vi "NE-50X Single Run Edited.vi"() -> ()   [LabVIEW 2020]
doc: "This VI allows to perform a single run pumping mode : the pump run continuously until the user decide to stop, reverse or pause it."
uses:
  <vilib>/Utility/error.llb/DialogType.ctl
panel:
  in  "Extrusions to Do":i32
  out "Extrusions":i32
  in  "Volume":dbl
  out "Firmware Version":string
  out "Firmware Version":string
  in  "Secondary Pump Address":i32 format="%0#.0f"
  in  "Master Pump Address":i32 format="%0#.0f"
  out "Tank 2":dbl(slide)
  out "x+y":i32
  out "Tank":dbl(slide)
  in  "PAUSE 2":bool
  in  "Baud Rate (19200)":u32(ring)=19200 items=["19200"=19200, "9600"=9600, "2400"=2400, "1200"=1200, "300"=300]
  in  "VISA resource name":refnum<visa-resource-name>="ASRL1::INSTR"
  in  "PAUSE":bool
  in  "RUN":bool
  in  "STOP":bool
  in  "Audible Alarms":bool=TRUE
  in  "Flow rate\nSee below to enter a right value for flow rate":dbl=0.5 format="%.3f"
  in  "Units":i32(ring) items=["microlitters per minute (µL/min)", "microlitters per hour (µL/hr)", "milliliters per minute (mL/min)", "milliliters per hour (mL/hr)"]
  in  "Initial Direction":u16(ring) items=["Infuse", "Withdraw"]
  in  "Syringe Inside Diameter (19.58 mm)\nIf diameter is upper than 14.00 mm : Volume units are mL\nIf diameter is lower than 14.00 mm : Volume units are µL":dbl=19.58 min=0.1 max=50.0 step=0.01 format="%#_4g"
  out "Status":T1
  out "Volume Dispense":string
  # "Current Status"
  # "Configuration Settings"
  # "Pump System Config"
  # "mm"
  # "RS-232 Setup"
  # "Pump Control"
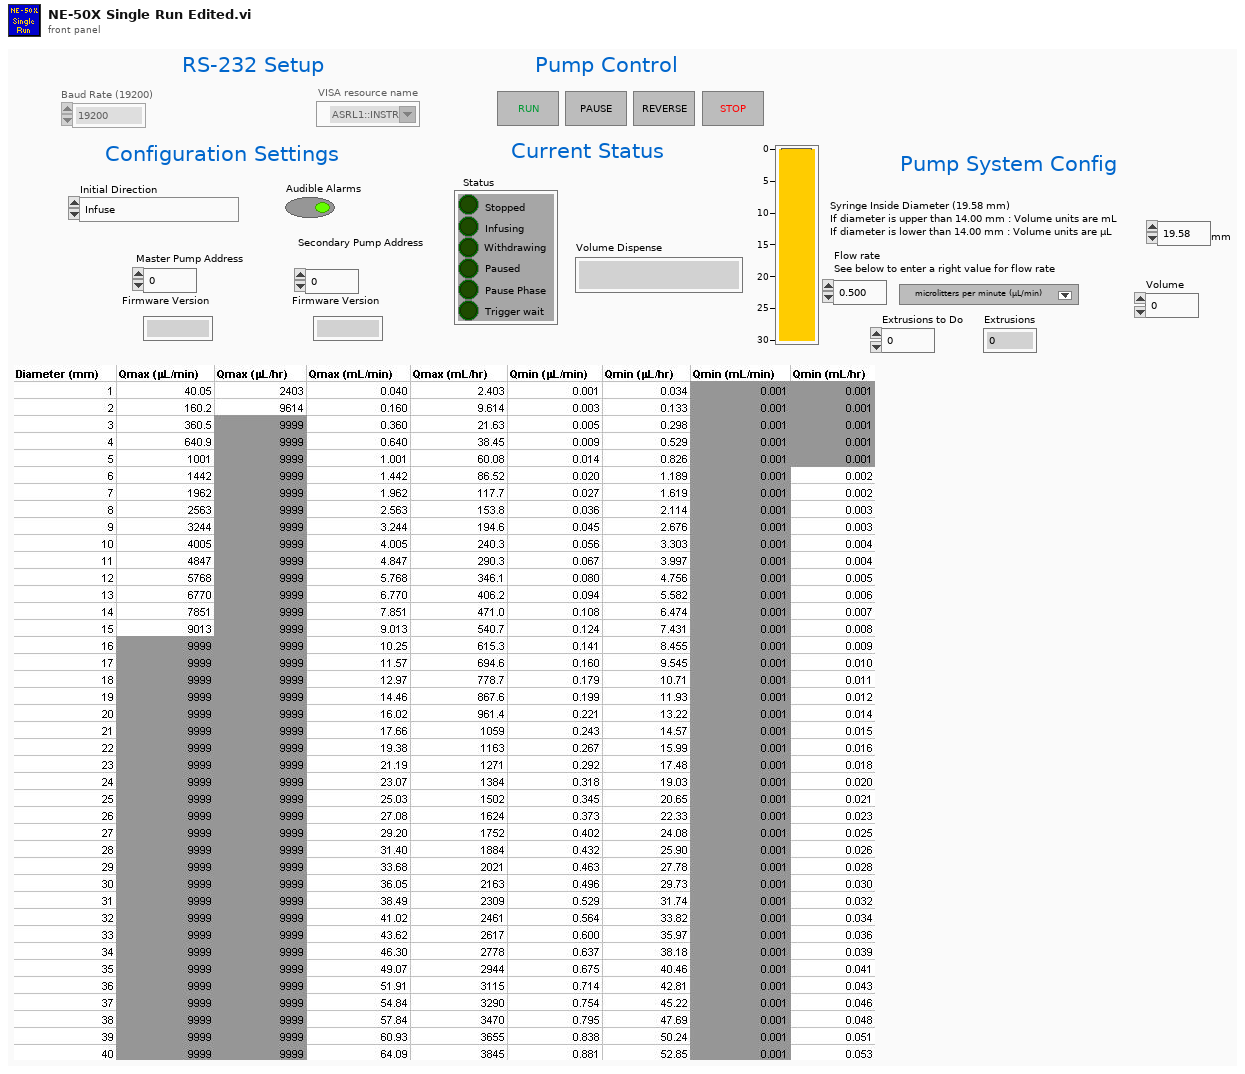
[diagram p1: front panel]
types:
  T1 = cluster{"Stopped":bool, "Infusing":bool, "Withdrawing":bool, "Paused":bool, "Pause Phase":bool, "Trigger wait":bool}
  T2 = typedef "DialogType.ctl" = u16
  T3 = cluster{"0=off\n1=on":u16, "Numbers of beeps\n0=continuously":dbl}
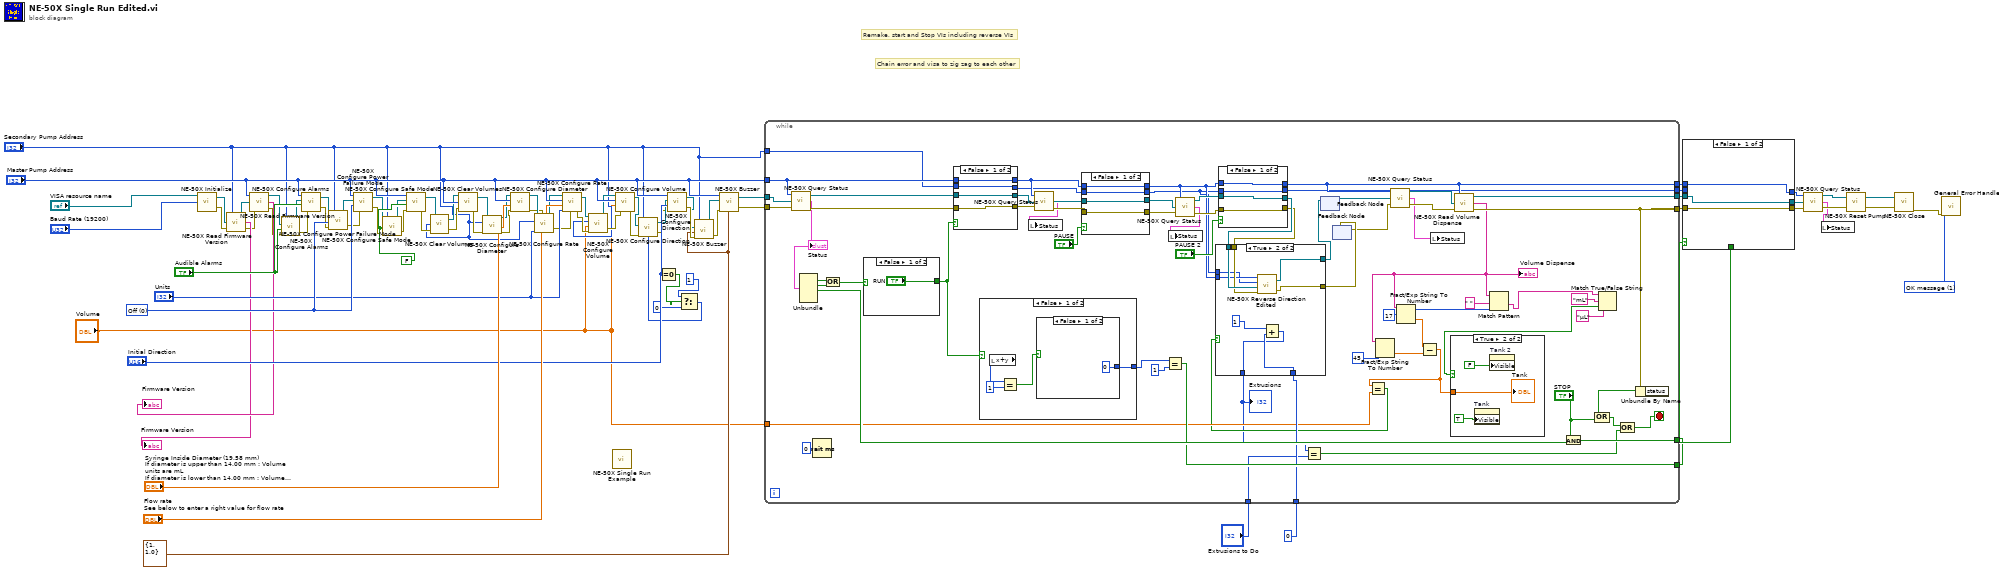
[diagram p0: block diagram]
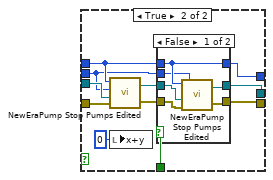
[diagram p2: hidden frame]
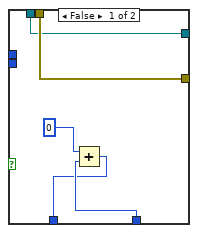
[diagram p4: hidden frame]
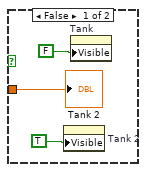
[diagram p5: hidden frame]
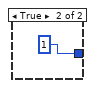
[diagram p6: hidden frame]
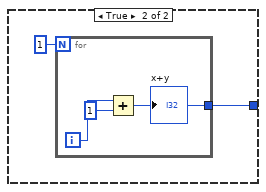
[diagram p7: hidden frame]
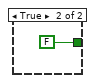
[diagram p8: hidden frame]
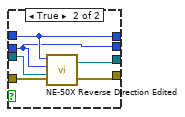
[diagram p9: hidden frame]
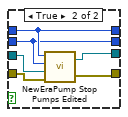
[diagram p10: hidden frame]
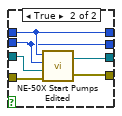
[diagram p11: hidden frame]
diagram:
  w62 = T2 1 items=["no dialog", "OK message", "continue or stop message", "OK message + warnings", "continue/stop + warnings"] ("type of dialog (OK msg:1)")
  w58 = FALSE ("0 = Basic")
  w59 = u16 0 items=["Off", "On"] ("0 = Disabled")
  w6 = T3 {"0=off\n1=on"=1, "Numbers of beeps\n0=continuously"=1.0} ("Buzzer")
  # "Chain error and visa to zig zag to each other"
  # "Remake, start and Stop VIs including reverse VIs"
  n1 = call <instrlib>:"NE-50X Initialize.vi"("Baud Rate (19200)"="Baud Rate (19200)", "VISA resource name"="VISA resource name") -> ("error out"=w48:errorcluster, "VISA resource name out"=w45:refnum<visa-resource-name>)  [unwired: 1 in]
  n2 = call <instrlib>:"NE-50X Read Firmware Version.vi"("error in (no error)"=w48, "VISA resource name"=w45, "Address (0)"="Secondary Pump Address") -> ("error out"=w43:errorcluster, "Version"=→"Firmware Version":string, "VISA resource name out"=w44:refnum<visa-resource-name>)
  n3 = call <instrlib>:"NE-50X Read Firmware Version.vi"("error in (no error)"=w43, "VISA resource name"=w44, "Address (0)"="Master Pump Address") -> ("error out"=w41:errorcluster, "Version"=→"Firmware Version":string, "VISA resource name out"=w42:refnum<visa-resource-name>)
  n4 = call <instrlib>:"NE-50X Configure Alarms.vi"("error in (no error)"=w41, "Audible Alarms"="Audible Alarms", "VISA resource name"=w42, "Address (0)"="Secondary Pump Address") -> ("error out"=w40:errorcluster, "VISA resource name out"=w39:refnum<visa-resource-name>)
  n5 = call <instrlib>:"NE-50X Configure Alarms.vi"("error in (no error)"=w40, "Audible Alarms"="Audible Alarms", "VISA resource name"=w39, "Address (0)"="Master Pump Address") -> ("error out"=w38:errorcluster, "VISA resource name out"=w37:refnum<visa-resource-name>)
  n6 = call <instrlib>:"NE-50X Configure Power Failure Mode.vi"("error in (no error)"=w38, "Power Failure Mode"=w59, "VISA resource name"=w37, "Address (0)"="Secondary Pump Address") -> ("error out"=w35:errorcluster, "VISA resource name out"=w36:refnum<visa-resource-name>)
  n7 = call <instrlib>:"NE-50X Configure Power Failure Mode.vi"("error in (no error)"=w35, "Power Failure Mode"=w59, "VISA resource name"=w36, "Address (0)"="Master Pump Address") -> ("error out"=w34:errorcluster, "VISA resource name out"=w31:refnum<visa-resource-name>)
  n8 = call <instrlib>:"NE-50X Configure Safe Mode.vi"("error in (no error)"=w34, "Safe Mode"=w58, "VISA resource name"=w31, "Address (0)"="Secondary Pump Address") -> ("error out"=w33:errorcluster, "VISA resource name out"=w32:refnum<visa-resource-name>)
  n9 = call <instrlib>:"NE-50X Configure Safe Mode.vi"("error in (no error)"=w33, "Safe Mode"=w58, "VISA resource name"=w32, "Address (0)"="Master Pump Address") -> ("error out"=w27:errorcluster, "VISA resource name out"=w30:refnum<visa-resource-name>)
  n10 = call <instrlib>:"NE-50X Clear Volumes.vi"("error in (no error)"=w27, "Address (0)"="Secondary Pump Address", "VISA resource name"=w30) -> ("error out"=w28:errorcluster, "VISA resource name out"=w29:refnum<visa-resource-name>)
  n11 = call <instrlib>:"NE-50X Clear Volumes.vi"("error in (no error)"=w28, "Address (0)"="Master Pump Address", "VISA resource name"=w29) -> ("error out"=w25:errorcluster, "VISA resource name out"=w26:refnum<visa-resource-name>)
  n12 = call <instrlib>:"NE-50X Configure Diameter.vi"("error in (no error)"=w25, "Diameter (19.58 mm)"="Syringe Inside Diameter (19.58 mm)\nIf diameter is upper than 14.00 mm : Volume units are mL\nIf diameter is lower than 14.00 mm : Volume units are µL", "Address (0)"="Secondary Pump Address", "VISA resource name"=w26) -> ("error out"=w23:errorcluster, "VISA resource name out"=w24:refnum<visa-resource-name>)  [unwired: 1 in, 1 out]
  n13 = call <instrlib>:"NE-50X Configure Diameter.vi"("error in (no error)"=w23, "Diameter (19.58 mm)"="Syringe Inside Diameter (19.58 mm)\nIf diameter is upper than 14.00 mm : Volume units are mL\nIf diameter is lower than 14.00 mm : Volume units are µL", "Address (0)"="Master Pump Address", "VISA resource name"=w24) -> ("error out"=w21:errorcluster, "VISA resource name out"=w22:refnum<visa-resource-name>)  [unwired: 1 in, 1 out]
  n14 = call <instrlib>:"NE-50X Configure Rate.vi"("VISA resource name"=w22, "Address (0)"="Secondary Pump Address", "Flow"="Flow rate\nSee below to enter a right value for flow rate", "Units"="Units", "error in (no error)"=w21) -> ("VISA resource name out"=w20:refnum<visa-resource-name>, "error out"=w19:errorcluster)
  n15 = call <instrlib>:"NE-50X Configure Rate.vi"("VISA resource name"=w20, "Address (0)"="Master Pump Address", "Flow"="Flow rate\nSee below to enter a right value for flow rate", "Units"="Units", "error in (no error)"=w19) -> ("VISA resource name out"=w18:refnum<visa-resource-name>, "error out"=w17:errorcluster)
  n16 = call <instrlib>:"NE-50X Configure Volume.vi"("error in (no error)"=w17, "Volume"="Volume", "Address (0)"="Secondary Pump Address", "VISA resource name"=w18) -> ("error out"=w15:errorcluster, "VISA resource name out"=w16:refnum<visa-resource-name>)
  n17 = call <instrlib>:"NE-50X Single Run Example.vi"() -> ()  [unwired: 1 in]
  n18 = call <instrlib>:"NE-50X Configure Volume.vi"("error in (no error)"=w15, "Volume"="Volume", "Address (0)"="Master Pump Address", "VISA resource name"=w16) -> ("error out"=w13:errorcluster, "VISA resource name out"=w14:refnum<visa-resource-name>)
  n19 = Equal To 0?(x="Initial Direction") -> (x = 0?=w53:bool)
  n20 = Select(t=1, s=w53, f=0) -> (s? t:f=w52:i32)
  n21 = call <instrlib>:"NE-50X Configure Direction.vi"("error in (no error)"=w13, "Direction"=w52, "VISA resource name"=w14, "Address (0)"="Secondary Pump Address") -> ("error out"=w11:errorcluster, "VISA resource name out"=w12:refnum<visa-resource-name>)
  n22 = call <instrlib>:"NE-50X Configure Direction.vi"("error in (no error)"=w11, "Direction"="Initial Direction", "VISA resource name"=w12, "Address (0)"="Master Pump Address") -> ("error out"=w10:errorcluster, "VISA resource name out"=w8:refnum<visa-resource-name>)
  n23 = call <instrlib>:"NE-50X Buzzer.vi"("error in (no error)"=w10, "Buzzer"=w6, "VISA resource name"=w8, "Address (0)"="Secondary Pump Address") -> ("error out"=w9:errorcluster, "VISA resource name out"=w7:refnum<visa-resource-name>)
  n24 = call <instrlib>:"NE-50X Buzzer.vi"("error in (no error)"=w9, "Buzzer"=w6, "VISA resource name"=w7, "Address (0)"="Master Pump Address") -> ("error out"=w49:errorcluster, "VISA resource name out"=w72:refnum<visa-resource-name>)
  n25 = while {
    tunnel: w72 -> [w121]
    tunnel: w49 -> [w146]
    tunnel: [w141] -> w70
    tunnel: [w140] -> w71
    tunnel: "Master Pump Address" -> [w120]
    tunnel: [w116] -> w69
    tunnel: [w111] -> w66
    tunnel: [w107] -> w64
    tunnel: "Secondary Pump Address" -> [w99]
    tunnel: [w97] -> w4
    tunnel: 0 -> [w96]
    tunnel: "Volume" -> [w94]
    tunnel: "Extrusions to Do" -> [w83]
    stop <- w80 stop-if-true
    n26 = call <instrlib>:"NE-50X Query Status.vi"("error in (no error)"=w146, "VISA resource name"=w121, "Address (0)"=w120) -> ("error out"=w143:errorcluster, "Status"=w135:T1, "VISA resource name out"=w144:refnum<visa-resource-name>)
    "Status" <- w135
    n27 = Unbundle(w135) -> ("Infusing"=w134:bool, "Withdrawing"=w133:bool, "Paused"=w112:bool)  [unwired: 3 out]
    n28 = Wait (ms)(milliseconds to wait=u32 0) -> ()  [unwired: 1 out]
    n29 = Or(x=w134, y=w133) -> (x .or. y?=w132:bool)
    n30 = case shown="False" w132 {
      tunnel: ["RUN" FALSE ("RUN")] -> w108
      frame False {
      }
      frame True {
      }
    }
    n31 = case shown="False" w108 {
      tunnel: w120 -> [w204 w206]
      tunnel: [w203 w207] -> w115
      tunnel: [w202 w208] -> w131
      tunnel: [w204 w206] -> w119
      tunnel: w144 -> [w203 w210]
      tunnel: w143 -> [w202 w209]
      tunnel: w99 -> [w201 w205]
      tunnel: [w201 w205] -> w98
      frame False {
      }
      frame True {
        n32 = call "NE-50X Start Pumps Edited.vi"("error in (no error)"=w209, "VISA resource name"=w210, "Secondary Pump Address (0)"=w205, "Master Pump Address (0)"=w206) -> ("error out"=w208:errorcluster, "VISA resource name out"=w207:refnum<visa-resource-name>)
      }
    }
    n33 = case shown="False" w108 {
      tunnel: [w168 w174] -> w110
      frame False {
        n34 = local read "x+y"() -> (w171:i32)
        n35 = Equal?(x=w171, y=1) -> (x = y?=w169:bool)
        n36 = case shown="False" w169 {
          tunnel: [0 1] -> w168
          frame False {
          }
          frame True {
          }
        }
      }
      frame True {
        n37 = for {
          N: 1 -> [_]
          tunnel: [w176] -> w174
          i -> [w178]
          n38 = Add(x=w178, y=1) -> (x+y=w176:i32)
          "x+y" <- w176
        }
      }
    }
    n39 = call <instrlib>:"NE-50X Query Status.vi"("error in (no error)"=w131, "VISA resource name"=w115, "Address (0)"=w119) -> ("error out"=w130:errorcluster, "Status"=w124:T1, "VISA resource name out"=w129:refnum<visa-resource-name>)
    n40 = local write "Status"(w124) -> ()
    n41 = case shown="False" "PAUSE" {
      tunnel: w119 -> [w194 w196]
      tunnel: w129 -> [w192 w200]
      tunnel: w130 -> [w193 w199]
      tunnel: [w193 w198] -> w128
      tunnel: [w192 w197] -> w118
      tunnel: [w194 w196] -> w86
      tunnel: w98 -> [w191 w195]
      tunnel: [w191 w195] -> w85
      frame False {
      }
      frame True {
        n42 = call "NewEraPump Stop Pumps Edited.vi"("error in (no error)"=w199, "VISA resource name"=w200, "Secondary Pump Address (0)"=w195, "Master Pump Address (0)"=w196) -> ("error out"=w198:errorcluster, "VISA resource name out"=w197:refnum<visa-resource-name>)
      }
    }
    n43 = Equal?(x=w110, y=1) -> (x = y?=w107:bool)
    n44 = call <instrlib>:"NE-50X Query Status.vi"("error in (no error)"=w128, "VISA resource name"=w118, "Address (0)"=w86) -> ("error out"=w126:errorcluster, "Status"=w123:T1, "VISA resource name out"=w127:refnum<visa-resource-name>)
    n45 = local write "Status"(w123) -> ()
    n46 = case shown="False" "PAUSE 2" {
      tunnel: w127 -> [w184 w190]
      tunnel: w86 -> [w182 w188]
      tunnel: [w184 w187] -> w92
      tunnel: [w183 w186] -> w91
      tunnel: w126 -> [w183 w189]
      tunnel: [w182 w188] -> w116
      tunnel: w85 -> [w181 w185]
      tunnel: [w181 w185] -> w97
      frame False {
      }
      frame True {
        n47 = call "NE-50X Reverse Direction Edited.vi"("error in (no error)"=w189, "VISA resource name"=w190, "Secondary Pump Address (0)"=w185, "Master Pump Address (0)"=w188) -> ("error out"=w186:errorcluster, "VISA resource name out"=w187:refnum<visa-resource-name>)
      }
    }
    n48 = feedback #1() -> (w89:refnum<visa-resource-name>)  [unwired: 1 in]
    n49 = feedback #2() -> (w87:errorcluster)  [unwired: 1 in]
    n50 = call <instrlib>:"NE-50X Query Status.vi"("error in (no error)"=w87, "VISA resource name"=w89, "Address (0)"=w116) -> ("error out"=w125:errorcluster, "Status"=w122:T1, "VISA resource name out"=w117:refnum<visa-resource-name>)
    n51 = local write "Status"(w122) -> ()
    n52 = call <instrlib>:"NE-50X Read Volume Dispense.vi"("error in (no error)"=w125, "VISA resource name"=w117, "Address (0)"=w116) -> ("error out"=w140:errorcluster, "Volume Dispense"=w106:string, "VISA resource name out"=w141:refnum<visa-resource-name>)
    "Volume Dispense" <- w106
    n53 = Fract/Exp String To Number(string=w106, offset=45) -> (number=w136:dbl)  [unwired: 2 in, 1 out]
    n54 = Fract/Exp String To Number(string=w106, offset=17) -> (offset past number=w104:i32, number=w137:dbl)  [unwired: 2 in]
    n55 = Subtract(x=w137, y=w136) -> (x-y=w95:dbl)
    n56 = Equal?(x=w95, y=w94) -> (x = y?=w93:bool)
    n57 = case shown="True" w93 {
      tunnel: w96 -> [w152 w161]
      tunnel: [w150 w159] -> w84
      tunnel: w92 -> [w148 w158]
      tunnel: w91 -> [w149 w157]
      tunnel: [w148 w156] -> w90
      tunnel: [w149 w155] -> w88
      tunnel: w86 -> [_ w154]
      tunnel: w85 -> [_ w153]
      frame False {
        n58 = Add(x=0, y=w152) -> (x+y=w150:i32)
      }
      frame True {
        n59 = call "NE-50X Reverse Direction Edited.vi"("error in (no error)"=w157, "VISA resource name"=w158, "Secondary Pump Address (0)"=w153, "Master Pump Address (0)"=w154) -> ("error out"=w155:errorcluster, "VISA resource name out"=w156:refnum<visa-resource-name>)
        n60 = Add(x=1, y=w161) -> (x+y=w159:i32)
      }
    }
    "Extrusions" <- w84
    n61 = Equal?(x=w84, y=w83) -> (x = y?=w82:bool)
    n62 = feedback-in #1(w90) -> ()
    n63 = feedback-in #2(w88) -> ()
    n64 = Match Pattern(string=w106, regular expression=" ", offset (0)=w104) -> (after substring=w100:string)  [unwired: 3 out]
    n65 = And(x="STOP", y=w112) -> (x .and. y?=w111:bool)
    n66 = Match True/False String(2:"µL" ("false string"), 3:"mL" ("true string"), 4:w100) -> (0:w101:bool)  [unwired: 1 out]
    n67 = case shown="True" w101 {
      tunnel: w95 -> [w163 w167]
      frame False {
        n68 = property on="Tank 2" class="Slide (strict)"("Visible"=TRUE) -> ()  [unwired: 2 in, 2 out]
        n69 = property on="Tank" class="Slide (strict)"("Visible"=FALSE) -> ()  [unwired: 2 in, 2 out]
        "Tank 2" <- w163
      }
      frame True {
        n70 = property on="Tank" class="Slide (strict)"("Visible"=TRUE) -> ()  [unwired: 2 in, 2 out]
        n71 = property on="Tank 2" class="Slide (strict)"("Visible"=FALSE) -> ()  [unwired: 2 in, 2 out]
        "Tank" <- w167
      }
    }
    n72 = Unbundle By Name(w140) -> ("status"=w114:bool)
    n73 = Compound Arithmetic op=OR(w114, "STOP") -> (w81:bool)
    n74 = Compound Arithmetic op=OR(w81, w82) -> (w80:bool)
  }
  n75 = case shown="False" w64 {
    tunnel: [w211 w224] -> w76
    tunnel: w71 -> [w211 w217]
    tunnel: w70 -> [w212 w218]
    tunnel: w69 -> [w213 w219]
    tunnel: [w212 w223] -> w68
    tunnel: w66 -> [_ w222]
    tunnel: [w213 w221] -> w65
    tunnel: w4 -> [_ w214]
    frame False {
    }
    frame True {
      n76 = call "NewEraPump Stop Pumps Edited.vi"("error in (no error)"=w217, "VISA resource name"=w218, "Secondary Pump Address (0)"=w214, "Master Pump Address (0)"=w219) -> ("error out"=w215:errorcluster, "VISA resource name out"=w216:refnum<visa-resource-name>)
      n77 = local write "x+y"(0 ("x+y")) -> ()
      n78 = case shown="False" w222 {
        tunnel: w215 -> [w227 w233]
        tunnel: [w225 w233] -> w224
        tunnel: w219 -> [w230 w231]
        tunnel: [w226 w232] -> w223
        tunnel: w216 -> [w228 w232]
        tunnel: [w230 w231] -> w221
        tunnel: w214 -> [w229 _]
        frame False {
          n79 = call "NewEraPump Stop Pumps Edited.vi"("error in (no error)"=w227, "VISA resource name"=w228, "Secondary Pump Address (0)"=w229, "Master Pump Address (0)"=w230) -> ("error out"=w225:errorcluster, "VISA resource name out"=w226:refnum<visa-resource-name>)
        }
        frame True {
        }
      }
    }
  }
  n80 = call <instrlib>:"NE-50X Query Status.vi"("error in (no error)"=w76, "VISA resource name"=w68, "Address (0)"=w65) -> ("error out"=w74:errorcluster, "Status"=w73:T1, "VISA resource name out"=w75:refnum<visa-resource-name>)
  n81 = local write "Status"(w73) -> ()
  n82 = call <instrlib>:"NE-50X Reset Pump.vi"("error in (no error)"=w74, "VISA resource name"=w75) -> ("error out"=w67:errorcluster, "VISA resource name out"=w78:refnum<visa-resource-name>)
  n83 = call <instrlib>:"NE-50X Close.vi"("VISA resource name"=w78, "error in (no error)"=w67) -> ("error out"=w63:errorcluster)  [unwired: 13 in]
  n84 = call <vilib>:"General Error Handler.vi"("type of dialog (OK msg:1)"=w62, "error in (no error)"=w63) -> ()  [unwired: 9 in, 5 out]
